vi "Name ini.vi"(6 "error in (no error)":errorcluster, 8 "Action":T1, 9 "Name in":string) -> (0 "error out":errorcluster, 2 "Name out":string)   [LabVIEW 2015]
uses:
  file/file action.ctl
  Calibration and Function folders.ctl
  <vilib>/Utility/config.llb/Write Key (String).vi
  <vilib>/Utility/config.llb/Read Key (String).vi
  <vilib>/Utility/config.llb/NI_LVConfig.lvlib
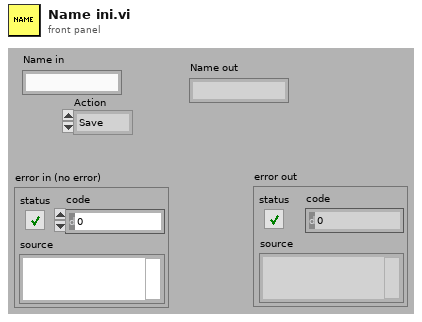
[diagram p1: front panel]
types:
  T1 = typedef "file action.ctl" = enum16{"Save", "Open"}
  T2 = typedef "Calibration and Function folders.ctl" = enum16{"Sensors", "Functions", "Config File", "PublicAppFolder", "New ini File", "Set Config File", "Delete ini File"}
  T3 = typedef "NI_LVConfig.lvlib/Config Data RefNum.ctl" = refnum<k1>
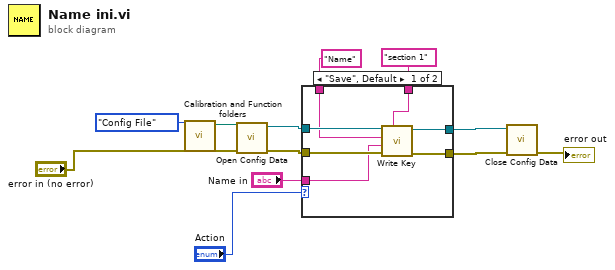
[diagram p0: block diagram]
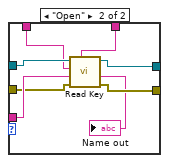
[diagram p2: hidden frame]
diagram:
  n1 = call "Calibration and Function folders.vi"("Folder"=Calibration_and_Function_folders."Config File") -> ("Selected Folder"=w4:path)  [unwired: 9 in, 1 out]
  n2 = call <vilib>:"Open Config Data.vi"("error in (no error)"="error in (no error)", "configuration file path"=w4) -> ("error out"=w12:errorcluster, "refnum"=w10:T3)  [unwired: 7 in, 1 out]
  n3 = case shown="\"Save\", Default" "Action" {
    tunnel: w12 -> [w19 w22]
    tunnel: [w18 w21] -> w11
    tunnel: w10 -> [w17 w27]
    tunnel: [w16 w26] -> w9
    tunnel: "section 1" ("section") -> [w15 w25]
    tunnel: "Name" ("key") -> [w14 w24]
    tunnel: "Name in" -> [w13 w23]
    frame "Save", Default {
      n4 = call-poly <vilib>:"Write Key.vi"("section"=w15, "error in (no error)"=w19, "value"=w13, "key"=w14, "refnum"=w17) -> ("error out"=w18:errorcluster, "refnum out"=w16:T3)  [unwired: 4 in, 1 out]
    }
    frame "Open" {
      n5 = call-poly <vilib>:"Read Key.vi"("section"=w25, "error in (no error)"=w22, "default value"=w23, "key"=w24, "refnum"=w27) -> ("error out"=w21:errorcluster, "value"=→"Name out":string, "refnum out"=w26:T3)  [unwired: 3 in, 1 out]
    }
  }
  n6 = call <vilib>:"Close Config Data.vi"("error in (no error)"=w11, "refnum"=w9) -> ("error out"=→"error out":errorcluster)  [unwired: 8 in, 1 out]
